vi "Launch Top Level Tasks.vi"(8 "error in (no error)":errorcluster, 11 "VolatusCoreTask in":refnum<class "VolatusCoreTask.lvclass">) -> (0 "error out":errorcluster, 3 "VolatusCoreTask out":refnum<class "VolatusCoreTask.lvclass">)   [LabVIEW 2020, in "Volatus.lvlib" / "VolatusCoreTask.lvclass"]
uses:
  VolatusCoreTask.lvclass
  VolatusCoreTask.lvclass/VolatusCoreTask.ctl
  Task/Task.lvclass
  C:/dev/lv20CE/relink/lv-volatus/Volatus/Task/Task.lvclass
  C:/Program Files (x86)/National Instruments/LabVIEW 2020/vi.lib/ActorFramework/Actor/Actor.lvclass
  C:/dev/lv20CE/relink/lv-volatus/Volatus/VolatusCoreTask/VolatusCoreTask.lvclass
  C:/dev/lv20CE/relink/lv-volatus/Volatus/APIRegistrationHandler/APIRegistrationHandler.lvclass
  C:/dev/lv20CE/relink/lv-volatus/Volatus/TaskStateHandler/TaskStateHandler.lvclass
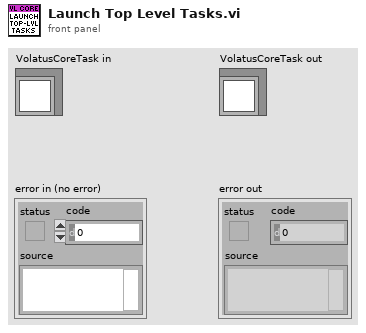
[diagram p1: front panel]
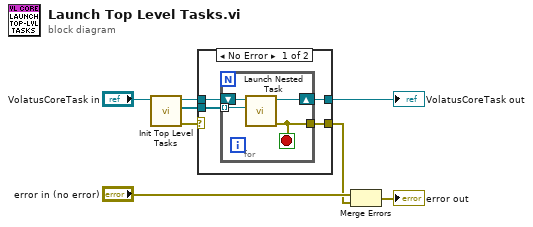
[diagram p0: block diagram]
diagram:
  n1 = call "Init Top Level Tasks.vi"("VolatusCoreTask in"="VolatusCoreTask in") -> ("error out"=w5:errorcluster, "Top Level Tasks"=w3:refnum<class "Task.lvclass">[], "VolatusCoreTask out"=w6:refnum<class "VolatusCoreTask.lvclass">)  [unwired: 8 in]
  n2 = case shown="No Error" w5 {
    selector: w5 -> [_ w18]
    tunnel: w6 -> [w12 w17]
    tunnel: [w9 w18] -> w1
    tunnel: [w10 w17] -> w4
    tunnel: w3 -> [w11 _]
    frame No Error {
      n3 = for {
        tunnel: w11 -> [w15] mode=indexing
        tunnel: [w14] -> w9
        shift-right: [w13] -> w10
        shift-left: w12 -> [w16]
        stop <- w14 stop-if-true
        n4 = call "Launch Nested Task.vi"("Nested Task"=w15, "Task in"=w16) -> ("error out"=w14:errorcluster, "Task out"=w13:refnum<class "VolatusCoreTask.lvclass">)  [unwired: 8 in]
      }
    }
    frame Error {
    }
  }
  "VolatusCoreTask out" <- w4
  n5 = Merge Errors("error in (no error)", w1) -> (→"error out":errorcluster)
